vi "SEQ Release Queue.vi"(8 "error in":errorcluster) -> (0 "error out":errorcluster)   [LabVIEW 2019, in "Allmotion.lvlib"]
uses:
  Allmotion.lvlib
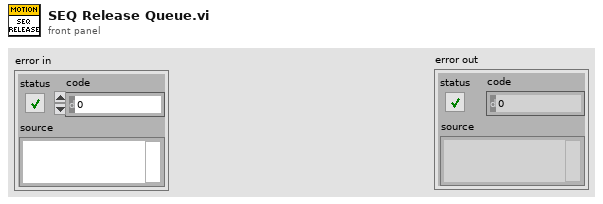
[diagram p1: front panel]
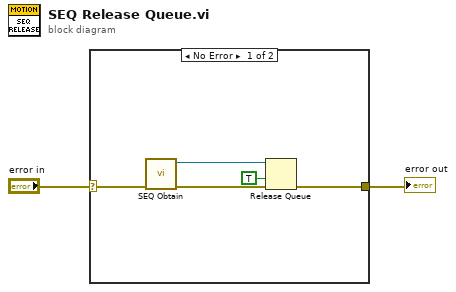
[diagram p0: block diagram]
diagram:
  n1 = case shown="No Error" "error in" {
    selector: "error in" -> [w7 w8]
    tunnel: [w3 w8] -> w1
    frame No Error {
      n2 = call "SEQ Obtain.vi"("error in"=w7) -> ("error out"=w6:errorcluster, "queue out"=w4:refnum<queue>)  [unwired: 9 in]
      n3 = Release Queue(queue=w4, force destroy? (F)=TRUE, error in (no error)=w6) -> (error out=w3:errorcluster)  [unwired: 2 out]
    }
    frame Error {
    }
  }
  "error out" <- w1
